vi "FTW-Endpoint-Multipart-Tell.vi"(0 "FTW Endpoint":refnum<class "FTW-Endpoint-TCP.lvclass">, 5 "Multipart Message":string[](array[string]), 7 "Timeout":i32 format="%dmsec", 11 "error in":errorcluster) -> (4 "FTW Endpoint out":refnum<class "FTW-Endpoint-TCP.lvclass">, 6 "Timed out?":bool, 15 "error out":errorcluster)   [LabVIEW 2013, in "FTW-Endpoint-TCP.lvclass"]
uses:
  FTW-Endpoint-TCP.lvclass
panel:
  # "Inputs"
  # "Outputs"
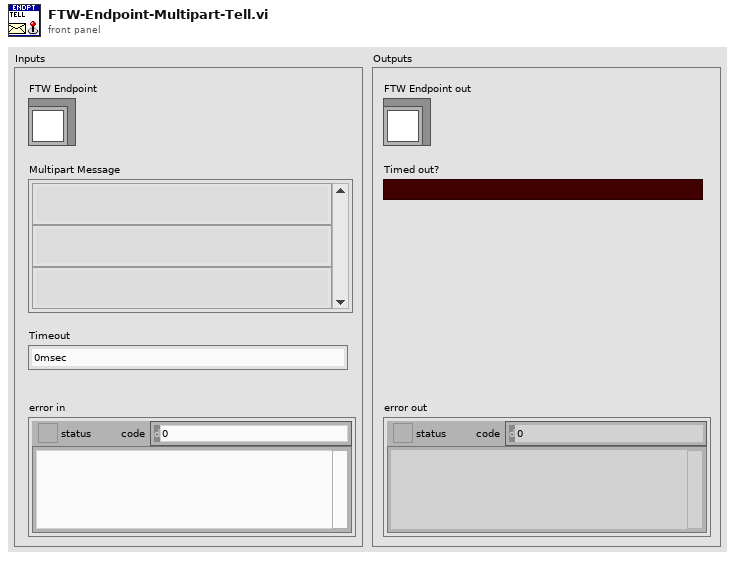
[diagram p1: front panel]
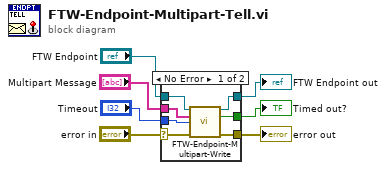
[diagram p0: block diagram]
diagram:
  n1 = case shown="No Error" "error in" {
    selector: "error in" -> [w14 w16]
    tunnel: [w13 w16] -> w7
    tunnel: [w11 w15] -> w5
    tunnel: "FTW Endpoint" -> [w12 w15]
    tunnel: "Multipart Message" -> [w10 _]
    tunnel: [w8 _] -> w2
    tunnel: "Timeout" -> [w9 _]
    frame No Error {
      n2 = call-dynamic "FTW-Endpoint-Multipart-Write.vi"("FTW Endpoint"=w12, "Multipart Message"=w10, "Timeout"=w9, "error in"=w14) -> ("FTW Endpoint out"=w11:refnum<class "FTW-Endpoint-TCP.lvclass">, "Timed out?"=w8:bool, "error out"=w13:errorcluster)  [unwired: 9 in]
    }
    frame Error {
    }
  }
  "error out" <- w7
  "FTW Endpoint out" <- w5
  "Timed out?" <- w2
